vi "Write States.vi"(8 "error in (no error)":errorcluster, 10 "States":T1, 11 "TestTactic in":refnum<class "TestTactic.lvclass">) -> (0 "error out":errorcluster, 3 "TestTactic out":refnum<class "TestTactic.lvclass">)   [LabVIEW 2023, in "TestTactic.lvclass"]
uses:
  TestTactic.lvclass
  States.ctl
  TestTactic.lvclass/TestTactic.ctl
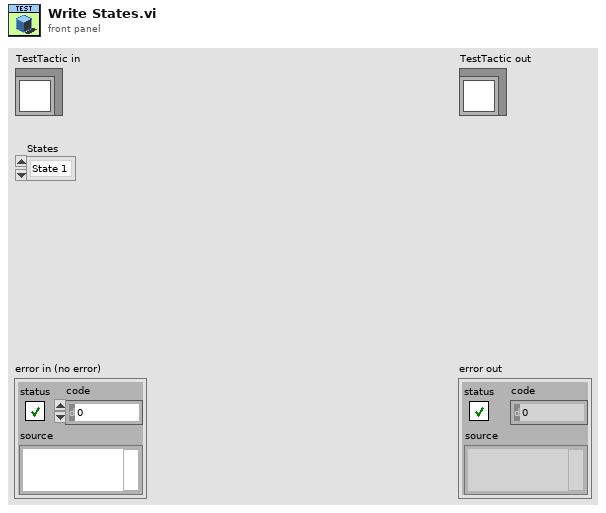
[diagram p1: front panel]
types:
  T1 = typedef "States.ctl" = enum16{"State 1", "Exit"}
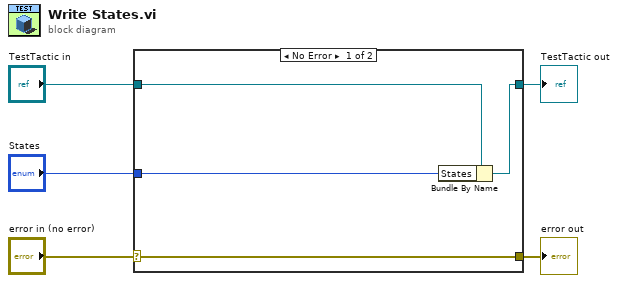
[diagram p0: block diagram]
diagram:
  n1 = case shown="No Error" "error in (no error)" {
    selector: "error in (no error)" -> [w9 w10]
    tunnel: [w9 w10] -> w4
    tunnel: [w7 w11] -> w2
    tunnel: "TestTactic in" -> [w8 w11]
    tunnel: "States" -> [w6 _]
    frame No Error {
      n2 = Bundle By Name(cluster=w8, "States"=w6) -> (w7:refnum<class "TestTactic.lvclass">)
    }
    frame Error {
    }
  }
  "error out" <- w4
  "TestTactic out" <- w2
